vi "SRV_Init_Comm_Loop.vi"(8 "error in (no error)":errorcluster, 10 "SRV IP Address":string) -> (0 "error out":errorcluster, 1 "Cancelled?":bool, 2 "SRV IP Address out":string, 3 "connection ID":refnum<k5>)   [LabVIEW 2009]
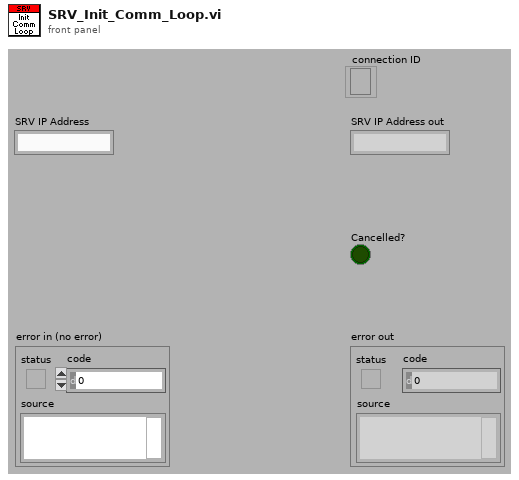
[diagram p1: front panel]
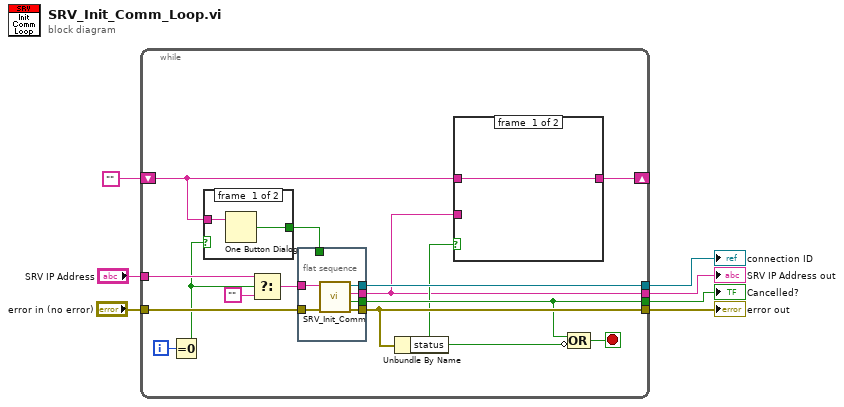
[diagram p0: block diagram]
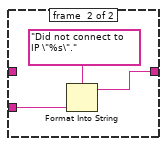
[diagram p3: hidden frame]
diagram:
  n1 = while {
    tunnel: [w20] -> w7
    tunnel: [w19] -> w6
    tunnel: [w12] -> w5
    tunnel: [w22] -> w4
    tunnel: "error in (no error)" -> [w21]
    tunnel: "SRV IP Address" -> [w16]
    shift-right: [w11] -> _
    shift-left: "" -> [w9]
    i -> [w17]
    stop <- w18 stop-if-true
    n2 = Equal To 0?(x=w17) -> (x = 0?=w10:bool)
    n3 = case shown="False" w10 {
      tunnel: w9 -> [w30 _]
      tunnel: [w29 _] -> w8
      frame #0 {
        n4 = One Button Dialog(message=w30) -> (true=w29:bool)  [unwired: 1 in]
      }
      frame #1 {
      }
    }
    n5 = Select(t=w16, s=w10, f="") -> (s? t:f=w15:string)
    n6 = flat-sequence {
      tunnel: [w28] -> w22
      tunnel: w21 -> [w27]
      tunnel: [w26] -> w20
      tunnel: [w25] -> w19
      tunnel: w15 -> [w24]
      tunnel: [w23] -> w12
      tunnel: w8 -> [_]
      frame #0 {
        n7 = call "SRV_Init_Comm.vi"("error in (no error)"=w27, "SRV IP Address"=w24) -> ("error out"=w26:errorcluster, "Cancelled?"=w25:bool, "SRV IP Address out"=w23:string, "connection ID"=w28:refnum<k5>)  [unwired: 6 in]
      }
    }
    n8 = Unbundle By Name(w20) -> ("status"=w13:bool)
    n9 = case shown="True" w13 {
      tunnel: w12 -> [_ w33]
      tunnel: [w31 w34] -> w11
      tunnel: w9 -> [w31 _]
      frame #0 {
      }
      frame #1 {
        n10 = Format Into String(format string="Did not connect to IP \"%s\".", w33) -> (resulting string=w34:string)  [unwired: 2 in, 1 out]
      }
    }
    n11 = Compound Arithmetic op=OR(w19, invert w13) -> (w18:bool)
  }
  "error out" <- w7
  "Cancelled?" <- w6
  "SRV IP Address out" <- w5
  "connection ID" <- w4
